vi "Send_single_wave.vi"(4 "error in (no error)":errorcluster, 6 "Amplitude":dbl, 7 "Max sample rate":dbl, 8 "Name":string, 9 "Cant. Freq":dbl, 10 "Frequency":dbl, 11 "VISA resource name":refnum<visa-resource-name>) -> (0 "error out":errorcluster, 3 "VISA resource name out":refnum<visa-resource-name>)   [LabVIEW 2018]
uses:
  <instrlib>/Tektronix AWG 5000 7000 Series/Tektronix AWG 5000 7000 Series.lvlib
panel:
  out "Waveform Graph":waveform(dbl)(graph)
  out "Samples":i32
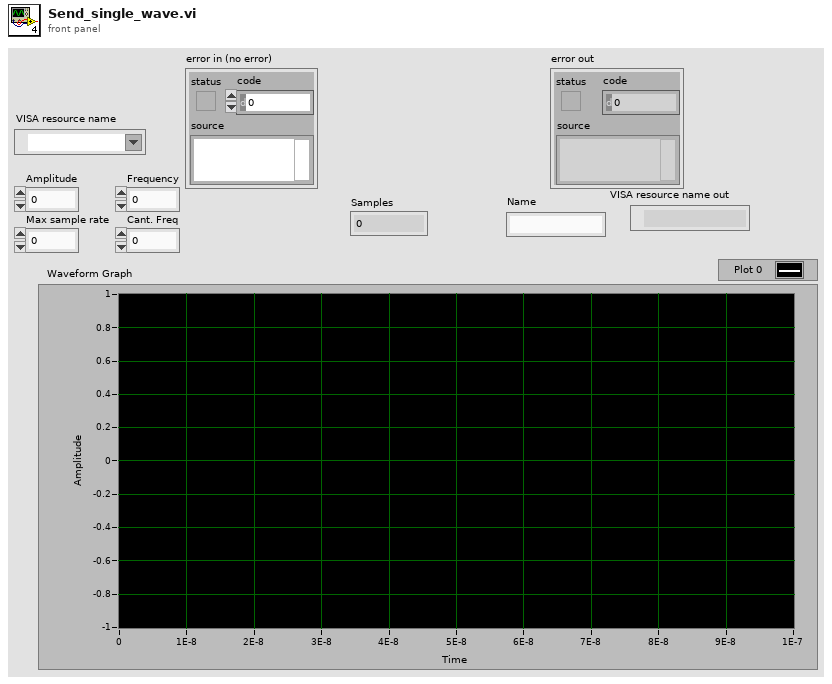
[diagram p1: front panel]
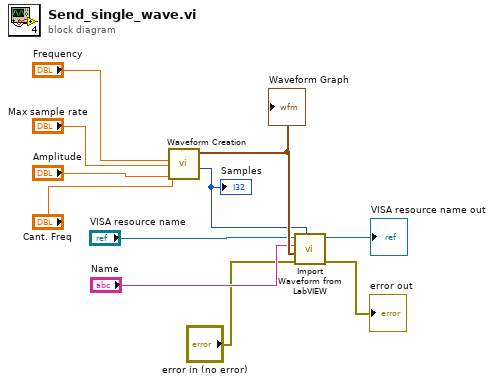
[diagram p0: block diagram]
diagram:
  n1 = call "Waveform Creation.vi"("Amplitude"="Amplitude", "Max sample rate"="Max sample rate", "Frequency"="Frequency", "Cant. Freq"="Cant. Freq") -> ("Samples"=w5:i32, "Waveform Graph"=w7:waveform(dbl))  [unwired: 6 in]
  "Samples" <- w5
  "Waveform Graph" <- w7
  n2 = call <instrlib>:"Import Waveform from LabVIEW.vi"("Sample Count (1000)"=w5, "error in (no error)"="error in (no error)", "Waveform"=w7, "Waveform Name"="Name", "VISA resource name"="VISA resource name") -> ("error out"=→"error out":errorcluster, "VISA resource name out"=→"VISA resource name out":refnum<visa-resource-name>)  [unwired: 5 in]
